vi "Launcher.vi"   [LabVIEW 2015]
uses:
  <vilib>/ActorFramework/Actor/Actor.lvclass
  Server/Server/Server.lvclass
panel:
  # "Actor Chat Window - Launcher!\nTom's LabVIEW Adventure\nhttps://www.youtube.com/tomslabviewadventure"
types:
  T1 = enum32{"Invalid", "Standard", "Closed", "Hidden", "Minimized", "Maximized"}
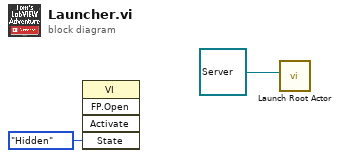
[diagram p0: block diagram]
diagram:
  n1 = invoke class="VI" method="FP.Open"("State"=T1."Hidden") -> ()  [unwired: 4 in, 5 out]
  n2 = call <vilib>:"Launch Root Actor.vi"("Actor"=refnum<class "Server.lvclass"> refnum ("Server.lvlib:Server.lvclass")) -> ()  [unwired: 9 in, 2 out]
